vi "test Remove Alias With Extra Empty Items.vi"(8 "error in (no error)":errorcluster, 11 "TestCase in":refnum<class "Routing and Faulting Aliases Unit Tests.lvclass">) -> (0 "error out":errorcluster, 3 "TestCase out":refnum<class "Routing and Faulting Aliases Unit Tests.lvclass">)   [LabVIEW 2019, in "Routing and Faulting Aliases Unit Tests.lvclass"]
uses:
  Routing and Faulting Aliases Unit Tests.lvclass
  System Explorer/Alias.ctl
  System Explorer/Endpoint.ctl
  Shared/Alias Endpoint.ctl
  Shared/Alias Mapping.ctl
  Routing and Faulting Aliases Unit Tests.lvclass/Routing and Faulting Aliases Unit Tests.ctl
  <vilib>/addons/_JKI Toolkits/VI Tester/TestCase.llb/TestCase.lvclass
  System Explorer/Routing and Faulting System Explorer.lvlib
  Scripting/Routing and Faulting Scripting.lvlib
  Shared/Routing and Faulting Shared.lvlib
  C:/Program Files (x86)/National Instruments/LabVIEW 2019/vi.lib/addons/_JKI Toolkits/VI Tester/TestCase.llb/TestCase.lvclass
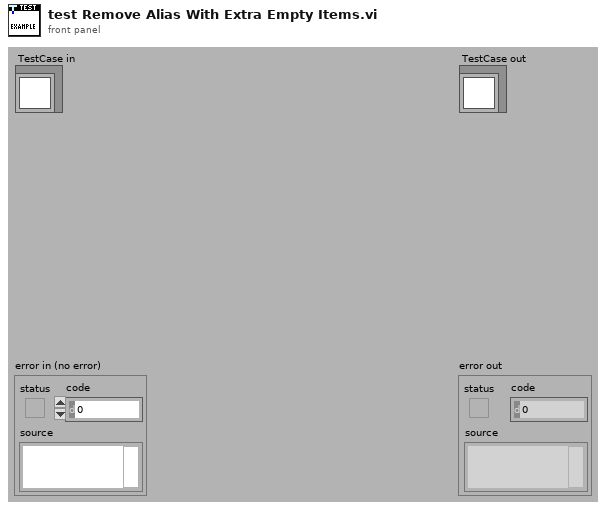
[diagram p1: front panel]
types:
  T1 = typedef "Routing and Faulting Shared.lvlib/Alias Mapping.ctl" = cluster{"Alias":string, "Endpoint":T2}
  T2 = typedef "Routing and Faulting Shared.lvlib/Alias Endpoint.ctl" = cluster{"Module Path":string, "Endpoint":string}
  T3 = typedef "Routing and Faulting System Explorer.lvlib/Endpoint.ctl" = string
  T4 = typedef "Routing and Faulting System Explorer.lvlib/Alias.ctl" = cluster{"Endpoint":T3, "Alias":string, "Remove":bool}
  T5 = typedef "Custom Device API.lvlib/Custom Device Item Ref.ctl" = u64
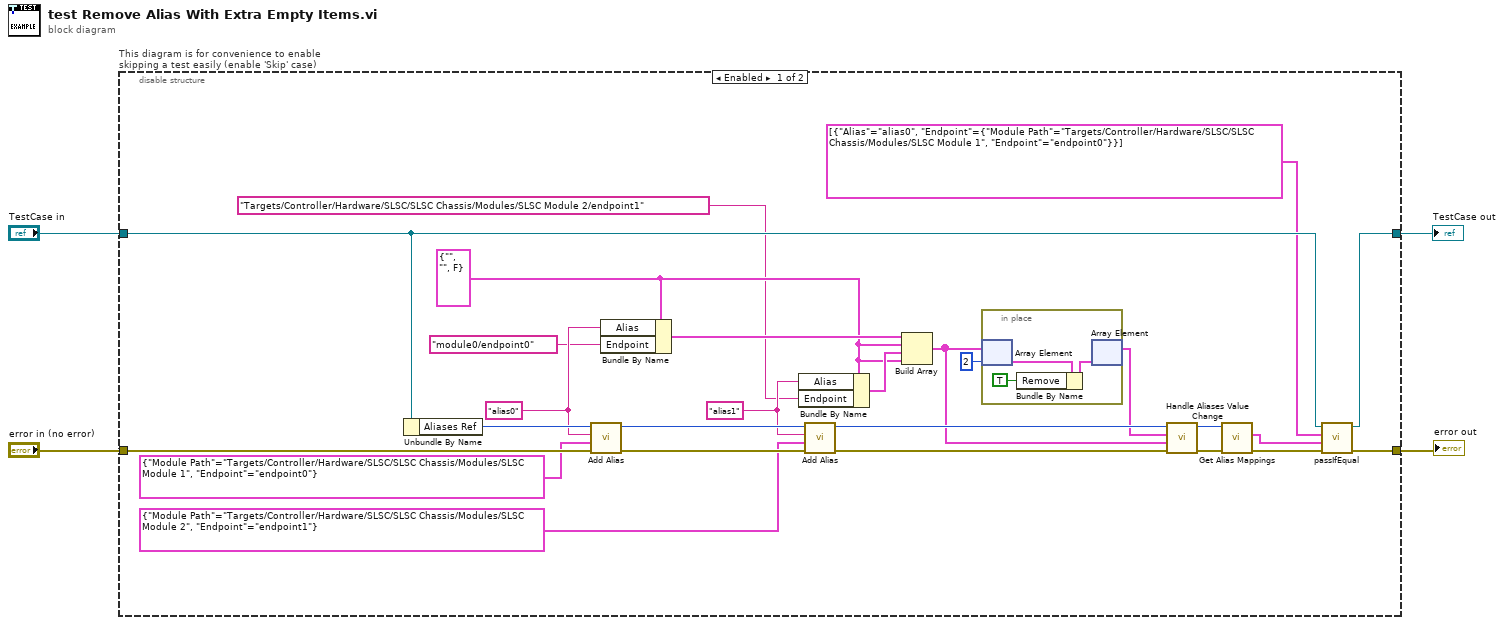
[diagram p0: block diagram]
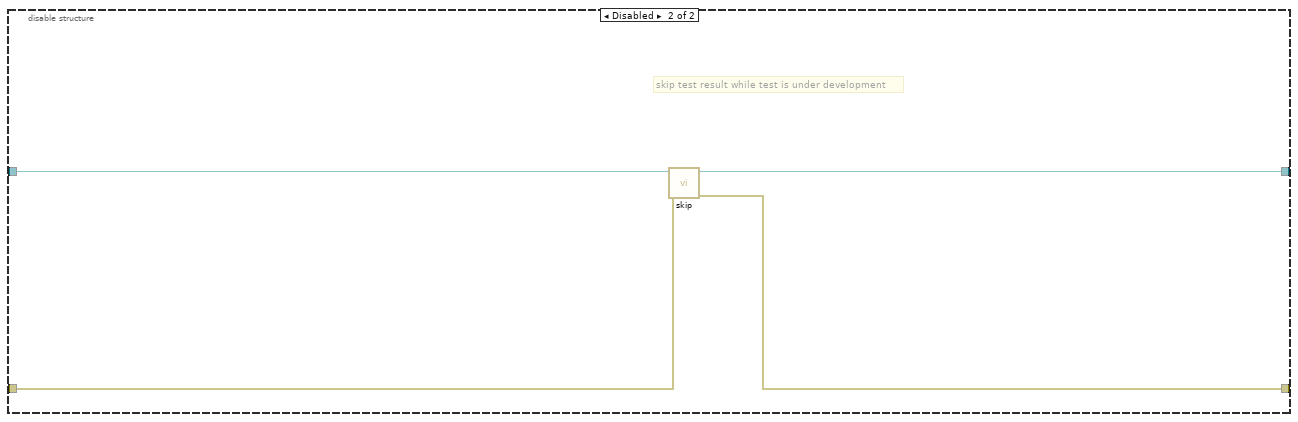
[diagram p2: hidden frame]
diagram:
  n1 = disable-structure "This diagram is for convenience to enable skipping a test easily (enable 'Skip' case)" shown="Enabled" {
    disable-tunnel: "TestCase in" -> [w25 w37]
    disable-tunnel: [w24 w35] -> w1
    disable-tunnel: [w27 w36] -> w3
    disable-tunnel: "error in (no error)" -> [w22 w34]
    frame Enabled {
      w15 = T4 {"Endpoint"="", "Alias"="", "Remove"=FALSE} ("Alias")
      w18 = "alias1" ("Alias")
      w19 = "alias0" ("Alias")
      n2 = Unbundle By Name(w25) -> ("Aliases Ref"=w23:T5)
      n3 = call "Add Alias.vi"("error in"=w22, "endpoint"=T2 {"Module Path"="Targets/Controller/Hardware/SLSC/SLSC Chassis/Modules/SLSC Module 1", "Endpoint"="endpoint0"} ("Endpoint"), "alias"=w19, "endpoint aliases in"=w23) -> ("error out"=w21:errorcluster, "endpoint aliases out"=w20:T5)  [unwired: 6 in]
      n4 = Bundle By Name(cluster=w15, "Alias"=w19, "Endpoint"=T3 "module0/endpoint0") -> (w17:T4)
      n5 = Bundle By Name(cluster=w15, "Alias"=w18, "Endpoint"=T3 "Targets/Controller/Hardware/SLSC/SLSC Chassis/Modules/SLSC Module 2/endpoint1") -> (w16:T4)
      n6 = call "Add Alias.vi"("error in"=w21, "endpoint"=T2 {"Module Path"="Targets/Controller/Hardware/SLSC/SLSC Chassis/Modules/SLSC Module 2", "Endpoint"="endpoint1"} ("Endpoint"), "alias"=w18, "endpoint aliases in"=w20) -> ("error out"=w13:errorcluster, "endpoint aliases out"=w12:T5)  [unwired: 6 in]
      n7 = Build Array(w17, w15, w16, w15) -> (w10:T4[])
      n8 = in-place {
        n9 = in-place-array #1(w10, 2) -> (w33:T4)
        n10 = Bundle By Name(cluster=w33, "Remove"=TRUE) -> (w31:T4)
        n11 = in-place-array #1(w31) -> (w11:T4[])  [unwired: 1 out]
      }
      n12 = call "Handle Aliases Value Change.vi"("error in (no error)"=w13, "OldVal"=w10, "NewVal"=w11, "Aliases Ref in"=w12) -> ("error out"=w30:errorcluster, "Aliases Ref out"=w29:T5)  [unwired: 4 in, 2 out]
      n13 = call "Get Alias Mappings.vi"("error in"=w30, "endpoint aliases in"=w29) -> ("error out"=w28:errorcluster, "alias mappings"=w26:T1[])  [unwired: 7 in, 1 out]
      n14 = call-dynamic "passIfEqual.vi"("error in (no error)"=w28, "y"=w26, "x"=T1[] [{"Alias"="alias0", "Endpoint"={"Module Path"="Targets/Controller/Hardware/SLSC/SLSC Chassis/Modules/SLSC Module 1", "Endpoint"="endpoint0"}}] ("Alias Mappings"), "TestCase in"=w25) -> ("error out"=w27:errorcluster, "TestCase out"=w24:refnum<class "Routing and Faulting Aliases Unit Tests.lvclass">)  [unwired: 6 in]
    }
    frame Disabled {
      # "skip test result while test is under development"
      n15 = call <vilib>:"skip.vi"("error in (no error)"=w34, "TestCase in"=w37) -> ("error out"=w36:errorcluster, "TestCase out"=w35:refnum<class "Routing and Faulting Aliases Unit Tests.lvclass">)  [unwired: 8 in]
    }
  }
  "error out" <- w3
  "TestCase out" <- w1
